vi "dfd_FXP MRate CIC Simu.vi"(6 "output phase":i32, 7 "init? (T)":bool, 8 "FXPMRateSimState in":T1, 10 "FXP CIC":T3={"mMRate_Structure"=enum."CIC", "mMRate_Mode"=0, "mMRate_Factor"=0, "mMRate_FIRParams"={"mMRate_FIR_H"=[], "mMRate_FIR_IsNyquist?"=FALSE, "mMRate_FIR_IsSymmetric?"=FALSE}, "mMRate_CICParams"={"mMRate_CIC_#Stage"=2, "mMRate_CIC_Lag"=1, "mMRate_CIC_Type"=enum."Lowpass"}, "mMRate_Order"=0, "mMRate_Version"="2.0", "mMRate_Comments"="", "mMRate_RationalFactor"={"mMRate_L"=-1, "mMRate_M"=-1}, "mMRate_Fs"=1.0, "mMRate_Quantized?"=FALSE, "mMRate_QFilterGain"=1.0, "mMRate_CoefWl"=16, "mMRate_Scaling"={"mMRate_ScaleByPowerOf2?"=FALSE, "mMRate_ScaleType"=enum."Time Domain 1-Norm"}, "mMRate_InputWl"=16, "mMRate_OutputWl"=16, "mMRate_OutputMode"=enum."Truncation", "mMRate_MultMode"=enum."Truncated", "mMRate_BitPruning"=FALSE, "mMRate_GainWl"=16, "mMRate_OutputFwl"=0, "mMRate_SumIwl"=0, "mMRate_InputIwl "=16, "mMRate_SumWl"=32, "mMRate_CoefIwl"=0} {"mMRate_SumWl" min=1 max=32 step=1; "mMRate_InputIwl" min=1 max=32 step=1; "mMRate_GainWl" min=1 max=32 step=1; "mMRate_OutputWl" min=1 max=32 step=1; "mMRate_InputWl" min=1 max=32 step=1; "mMRate_CoefWl" min=1 max=32 step=1; "mMRate_Mode" items=["Default"=-1, "No Rate Change"=0, "Interpolation"=1, "Decimation"=2, "Interpolated"=3, "Rational"=4]}, 11 "signal in":i32[](array[numeric])) -> (0 "FXPMRateSimState out":T1, 3 "signal out":i32[](array[numeric]))   [LabVIEW 2017, in "NI_DigFilter_FXP.lvlib"]
uses:
  <vilib>/addons/Digital Filter Design/NI_DigFilter_FXP.lvlib
  <vilib>/addons/Digital Filter Design/_Objects.llb/DFD Multirate Filter Obj.ctl
  <vilib>/addons/Digital Filter Design/_Objects.llb/DFD Multirate Mode.ctl
  <vilib>/addons/Digital Filter Design/_Objects.llb/DFD Coef Norm Type.ctl
  <vilib>/addons/Digital Filter Design/_Objects.llb/DFD Round-off Mode.ctl
  <vilib>/addons/Digital Filter Design/_Objects.llb/DFD FXP MRate Multiply Mode.ctl
  <vilib>/addons/Digital Filter Design/_Objects.llb/dfd_FXP MRate Simu State.ctl
  <vilib>/addons/Digital Filter Design/_Objects.llb/dfd_Integer I160.ctl
  <vilib>/addons/Digital Filter Design/NI_DigFilterLicensed.lvlib
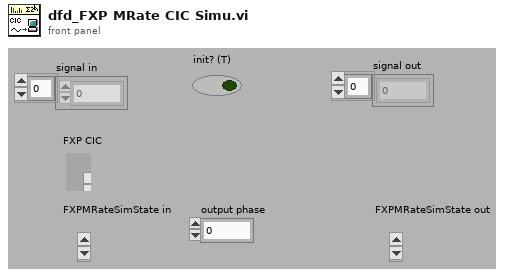
[diagram p1: front panel]
types:
  T1 = typedef "dfd_FXP MRate Simu State.ctl" = cluster{"acc1":T2[], "acc2":T2[], "FIR state":i64[], "next phase":i32}
  T2 = typedef "dfd_Integer I160.ctl" = cluster{"Hi [I32]":i32, "Lo3 [U32]":u32, "Lo2 [U32]":u32, "Lo1 [U32]":u32, "Lo0 [U32]":u32}
  T3 = typedef "NI_DigFilterLicensed.lvlib/DFD Multirate Filter Obj.ctl" = cluster{"mMRate_Structure":enum16{"CIC", "FIR", "IIR", "Lattice"}, "mMRate_Mode":T4, "mMRate_Factor":i32, "mMRate_FIRParams":cluster{"mMRate_FIR_H":dbl[], "mMRate_FIR_IsNyquist?":bool, "mMRate_FIR_IsSymmetric?":bool}, "mMRate_CICParams":cluster{"mMRate_CIC_#Stage":i32, "mMRate_CIC_Lag":i32, "mMRate_CIC_Type":enum16{"Lowpass", "Highpass"}}, "mMRate_Order":i32, "mMRate_Version":string, "mMRate_Comments":string, "mMRate_RationalFactor":cluster{"mMRate_L":i32, "mMRate_M":i32}, "mMRate_Fs":dbl, "mMRate_Quantized?":bool, "mMRate_QFilterGain":dbl, "mMRate_CoefWl":i16, "mMRate_Scaling":cluster{"mMRate_ScaleByPowerOf2?":bool, "mMRate_ScaleType":T5}, "mMRate_InputWl":i16, "mMRate_OutputWl":i16, "mMRate_OutputMode":T6, "mMRate_MultMode":T7, "mMRate_BitPruning":bool, "mMRate_GainWl":i16, "mMRate_OutputFwl":i16, "mMRate_SumIwl":i16, "mMRate_InputIwl ":i16, "mMRate_SumWl":i16, "mMRate_CoefIwl":i16}
  T4 = typedef "NI_DigFilterLicensed.lvlib/DFD Multirate Mode.ctl" = i16
  T5 = typedef "NI_DigFilterLicensed.lvlib/DFD Coef Norm Type.ctl" = enum16{"No Norm", "Time Domain 1-Norm", "Time Domain 2-Norm", "Time Domain Inf-Norm"}
  T6 = typedef "NI_DigFilterLicensed.lvlib/DFD Round-off Mode.ctl" = enum16{"Nearest", "Truncation"}
  T7 = typedef "NI_DigFilterLicensed.lvlib/DFD FXP MRate Multiply Mode.ctl" = enum16{"Truncated", "Full"}
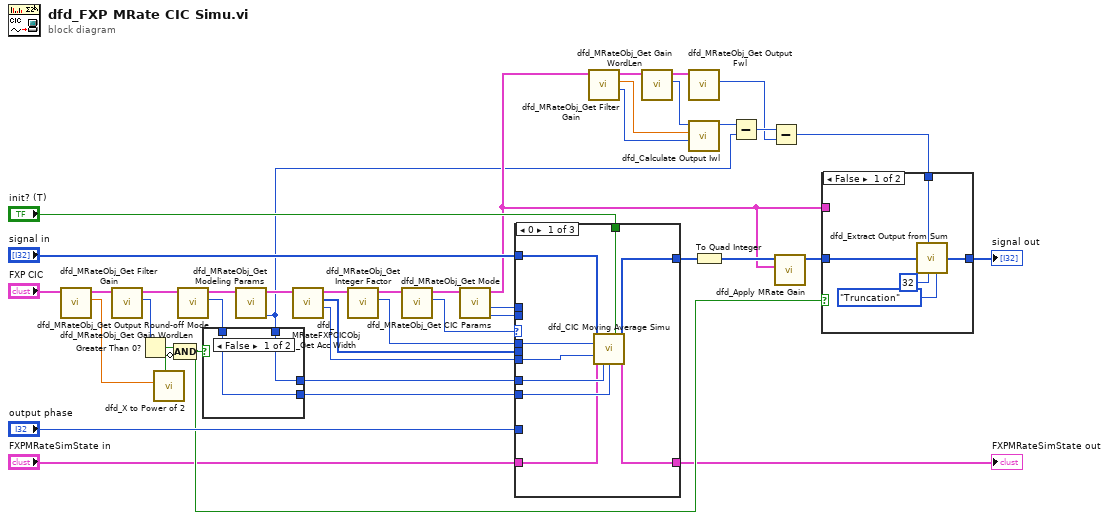
[diagram p0: block diagram]
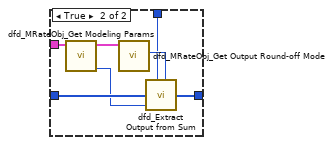
[diagram p2: hidden frame]
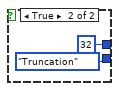
[diagram p3: hidden frame]
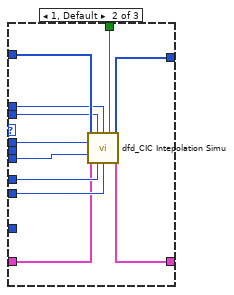
[diagram p4: hidden frame]
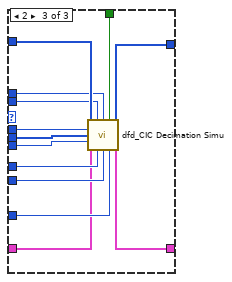
[diagram p5: hidden frame]
diagram:
  n1 = call <vilib>:"dfd_MRateObj_Get Filter Gain.vi"("multirate filter in"="FXP CIC") -> ("gain"=w35:dbl, "dup multirate filter"=w38:T3)  [unwired: 9 out]
  n2 = call <vilib>:"dfd_MRateObj_Get Gain WordLen.vi"("multirate filter in"=w38) -> ("gain wl"=w36:i16, "dup multirate filter"=w30:T3)  [unwired: 9 out]
  n3 = Greater Than 0?(x=w36) -> (x > 0?=w33:bool)
  n4 = call <vilib>:"dfd_X to Power of 2.vi"("x"=w35) -> ("is 2^n?"=w34:bool)  [unwired: 10 out]
  n5 = Compound Arithmetic op=AND(w33, invert w34) -> (w17:bool)
  n6 = call <vilib>:"dfd_MRateObj_Get Output Round-off Mode.vi"("multirate filter in"=w30) -> ("output round-off mode"=w29:T6, "dup multirate filter"=w21:T3)  [unwired: 9 out]
  n7 = call <vilib>:"dfd_MRateObj_Get Modeling Params.vi"("multirate filter in"=w21) -> ("output wl"=w1:i16, "dup multirate filter"=w20:T3)  [unwired: 9 out]
  n8 = case shown="False" w17 {
    tunnel: w29 -> [w44 _]
    tunnel: [w44 DFD_Round-off_Mode."Truncation" ("output round-off mode")] -> w32
    tunnel: w1 -> [w43 _]
    tunnel: [w43 i16 32 ("output wl")] -> w31
    frame False {
    }
    frame True {
    }
  }
  n9 = call <vilib>:"dfd_MRateFXPCICObj_Get Acc Width.vi"("FXP CIC in"=w20) -> ("MSB pos"=w39:i16, "Acc width"=w40:i32[], "dup FXP CIC"=w24:T3)  [unwired: 8 out]
  n10 = call <vilib>:"dfd_MRateObj_Get Integer Factor.vi"("multirate filter in"=w24) -> ("factor"=w23:i32, "dup multirate filter"=w26:T3)  [unwired: 9 out]
  n11 = call <vilib>:"dfd_MRateObj_Get Mode.vi"("multirate filter in"=w26) -> ("mode"=w25:T4, "dup multirate filter"=w22:T3)  [unwired: 9 out]
  n12 = call <vilib>:"dfd_MRateObj_Get CIC Params.vi"("multirate filter in"=w22) -> ("lag"=w27:i32, "# stages"=w28:i32, "dup multirate filter"=w3:T3)  [unwired: 8 out]
  n13 = case shown="0" w25 {
    tunnel: "signal in" -> [w50 w66 w79]
    tunnel: [w51 w65 w78] -> w13
    tunnel: "output phase" -> [_ _ w77]
    tunnel: w31 -> [w55 w64 w76]
    tunnel: w39 -> [w49 w63 w75]
    tunnel: w23 -> [w52 w62 w74]
    tunnel: w27 -> [_ w61 w73]
    tunnel: w28 -> [_ w60 w72]
    tunnel: w32 -> [w54 w59 w71]
    tunnel: w40 -> [_ _ w70]
    tunnel: "FXPMRateSimState in" -> [w48 w58 w69]
    tunnel: [w47 w57 w68] -> w15
    tunnel: "init? (T)" -> [w53 w56 w67]
    frame 0 {
      n14 = call <vilib>:"dfd_CIC Moving Average Simu.vi"("signal in"=w50, "init? (T)"=w53, "factor"=w52, "Output MSB pos"=w49, "FXPMRateSimState in"=w48, "Output wl"=w55, "q_mode"=w54) -> ("signal out"=w51:i32[], "FXPMRateSimState out"=w47:T1)  [unwired: 7 out]
    }
    frame 1, Default {
      n15 = call <vilib>:"dfd_CIC Intepolation Simu.vi"("signal in"=w66, "lag"=w61, "#stage"=w60, "init? (T)"=w56, "factor"=w62, "Output MSB pos"=w63, "FXPMRateSimState in"=w58, "Output wl"=w64, "q_mode"=w59) -> ("signal out"=w65:i32[], "FXPMRateSimState out"=w57:T1)  [unwired: 5 out]
    }
    frame 2 {
      n16 = call <vilib>:"dfd_CIC Decimation Simu.vi"("signal in"=w79, "lag"=w73, "#stage"=w72, "init? (T)"=w67, "factor"=w74, "Acc width"=w70, "MSB pos"=w75, "FXPMRateSimState in"=w69, "Output wl"=w76, "q_mode"=w71, "phase"=w77) -> ("signal out"=w78:i32[], "FXPMRateSimState out"=w68:T1)  [unwired: 3 out]
    }
  }
  "FXPMRateSimState out" <- w15
  n17 = call <vilib>:"dfd_MRateObj_Get Filter Gain.vi"("multirate filter in"=w3) -> ("sum iwl"=w9:i16, "gain"=w10:dbl, "dup multirate filter"=w11:T3)  [unwired: 8 out]
  n18 = call <vilib>:"dfd_MRateObj_Get Gain WordLen.vi"("multirate filter in"=w11) -> ("gain wl"=w7:i16, "dup multirate filter"=w6:T3)  [unwired: 9 out]
  n19 = call <vilib>:"dfd_MRateObj_Get Output Fwl.vi"("multirate filter in"=w6) -> ("output fwl"=w4:i16)  [unwired: 9 in, 1 out]
  n20 = call <vilib>:"dfd_Calculate Output Iwl.vi"("sum iwl"=w9, "gain value"=w10, "gain wl"=w7) -> ("output iwl"=w8:i16)  [unwired: 8 out]
  n21 = To Quad Integer(1:w13) -> (0:w12:i64[])
  n22 = Subtract(x=w8, y=w1) -> (x-y=w5:i16)
  n23 = Subtract(x=w5, y=w4) -> (x-y=w2:i16)
  n24 = call <vilib>:"dfd_Apply MRate Gain.vi"("multirate filter"=w3, "signal in"=w12) -> ("signal out"=w19:i64[])  [unwired: 1 in, 8 out]
  n25 = case shown="False" w17 {
    tunnel: w19 -> [w84 w91]
    tunnel: [w83 w90] -> w18
    tunnel: w3 -> [_ w89]
    tunnel: w2 -> [w82 w85]
    frame False {
      n26 = call <vilib>:"dfd_Extract Output from Sum.vi"("output iwl diff"=w82, "x"=w84, "output wl"=i16 32, "q_mode"=DFD_Round-off_Mode."Truncation") -> ("y"=w83:i32[])  [unwired: 5 out]
    }
    frame True {
      n27 = call <vilib>:"dfd_MRateObj_Get Modeling Params.vi"("multirate filter in"=w89) -> ("output wl"=w86:i16, "dup multirate filter"=w88:T3)  [unwired: 9 out]
      n28 = call <vilib>:"dfd_MRateObj_Get Output Round-off Mode.vi"("multirate filter in"=w88) -> ("output round-off mode"=w87:T6)  [unwired: 10 out]
      n29 = call <vilib>:"dfd_Extract Output from Sum.vi"("output iwl diff"=w85, "x"=w91, "output wl"=w86, "q_mode"=w87) -> ("y"=w90:i32[])  [unwired: 5 out]
    }
  }
  "signal out" <- w18
